vi "Teleop.vi"(10 "Match Info":T1={"Autonomous Elapsed Seconds"=0.0, "TeleOp Elapsed Seconds"=0.0, "Disabled Elapsed Seconds"=0.0, "Visited Autonomous"=FALSE, "Visited TeleOp"=FALSE, "Visited Disabled"=FALSE, "Autonomous Settings"={"Autonomous Style"=enum."Independent", "VI Refnum"=refnum}}, 11 "Call Context":T2) -> ()   [LabVIEW 2020]
doc: "This VI is called for each enabled TeleOp packet received from the DS. It is typically used to read from joysticks and other inputs and update I/O or setpoints for timed control loops. It should complete and return within 20 milliseconds or risk missing DS packets."
uses:
  <vilib>/Rock Robotics/Network Tables/NT Write Boolean Array.vi
  <vilib>/Rock Robotics/Network Tables/NT Write Numeric Array.vi
  Framework/Robot Global Data.vi
  <vilib>/Rock Robotics/WPI/DriverStation/WPI_DriverStationMatch Info.ctl
  <vilib>/Rock Robotics/WPI/DriverStation/WPI_DriverStationDerivedRobotMode.ctl
panel:
  in  "Duration(s)":dbl=3.0 format="%#_13g"
  in  "Shorter Setpoint":dbl=0.8 format="%#_13g"
  in  "Duration(s)":dbl=3.0 format="%#_13g"
  in  "Shorter Setpoint":dbl=0.8 format="%#_13g"
  in  "Duration(s)":dbl=3.0 format="%#_13g"
  in  "Shorter Setpoint":dbl=0.8 format="%#_13g"
  in  "Duration(s)":dbl=3.0 format="%#_13g"
  in  "Shorter Setpoint":dbl=0.8 format="%#_13g"
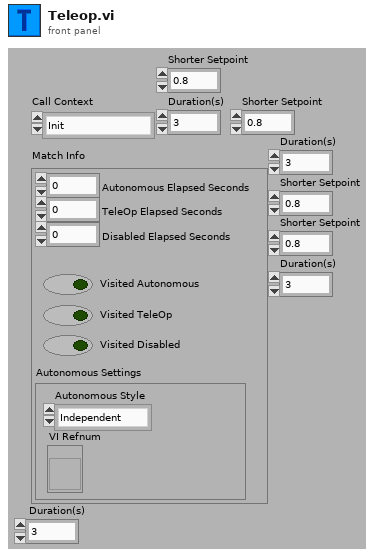
[diagram p1: front panel]
types:
  T1 = typedef "WPI_DriverStationMatch Info.ctl" = cluster{"Autonomous Elapsed Seconds":dbl, "TeleOp Elapsed Seconds":dbl, "Disabled Elapsed Seconds":dbl, "Visited Autonomous":bool, "Visited TeleOp":bool, "Visited Disabled":bool, "Autonomous Settings":cluster{"Autonomous Style":enum16{"Iterative", "Independent"}, "VI Refnum":refnum<vi>}}
  T2 = typedef "WPI_DriverStationDerivedRobotMode.ctl" = enum16{"Init", "Execute", "Stop"}
  T3 = typedef "WPI_JoystickDevRef.ctl" = cluster{"Device":T4}
  T4 = typedef "WPI_JoystickDeviceEnum.ctl" = enum16{"USB 0", "USB 1", "USB 2", "USB 3", "USB 4", "USB 5"}
  T5 = typedef "Command Status Info.ctl" = cluster{"Name":string, "Status":T6, "notifier out":T7}
  T6 = typedef "Completion Status.ctl" = enum16{"Successful", "Aborted", "Incomplete"}
  T7 = typedef "Completion Notifier.ctl" = refnum<notifier>
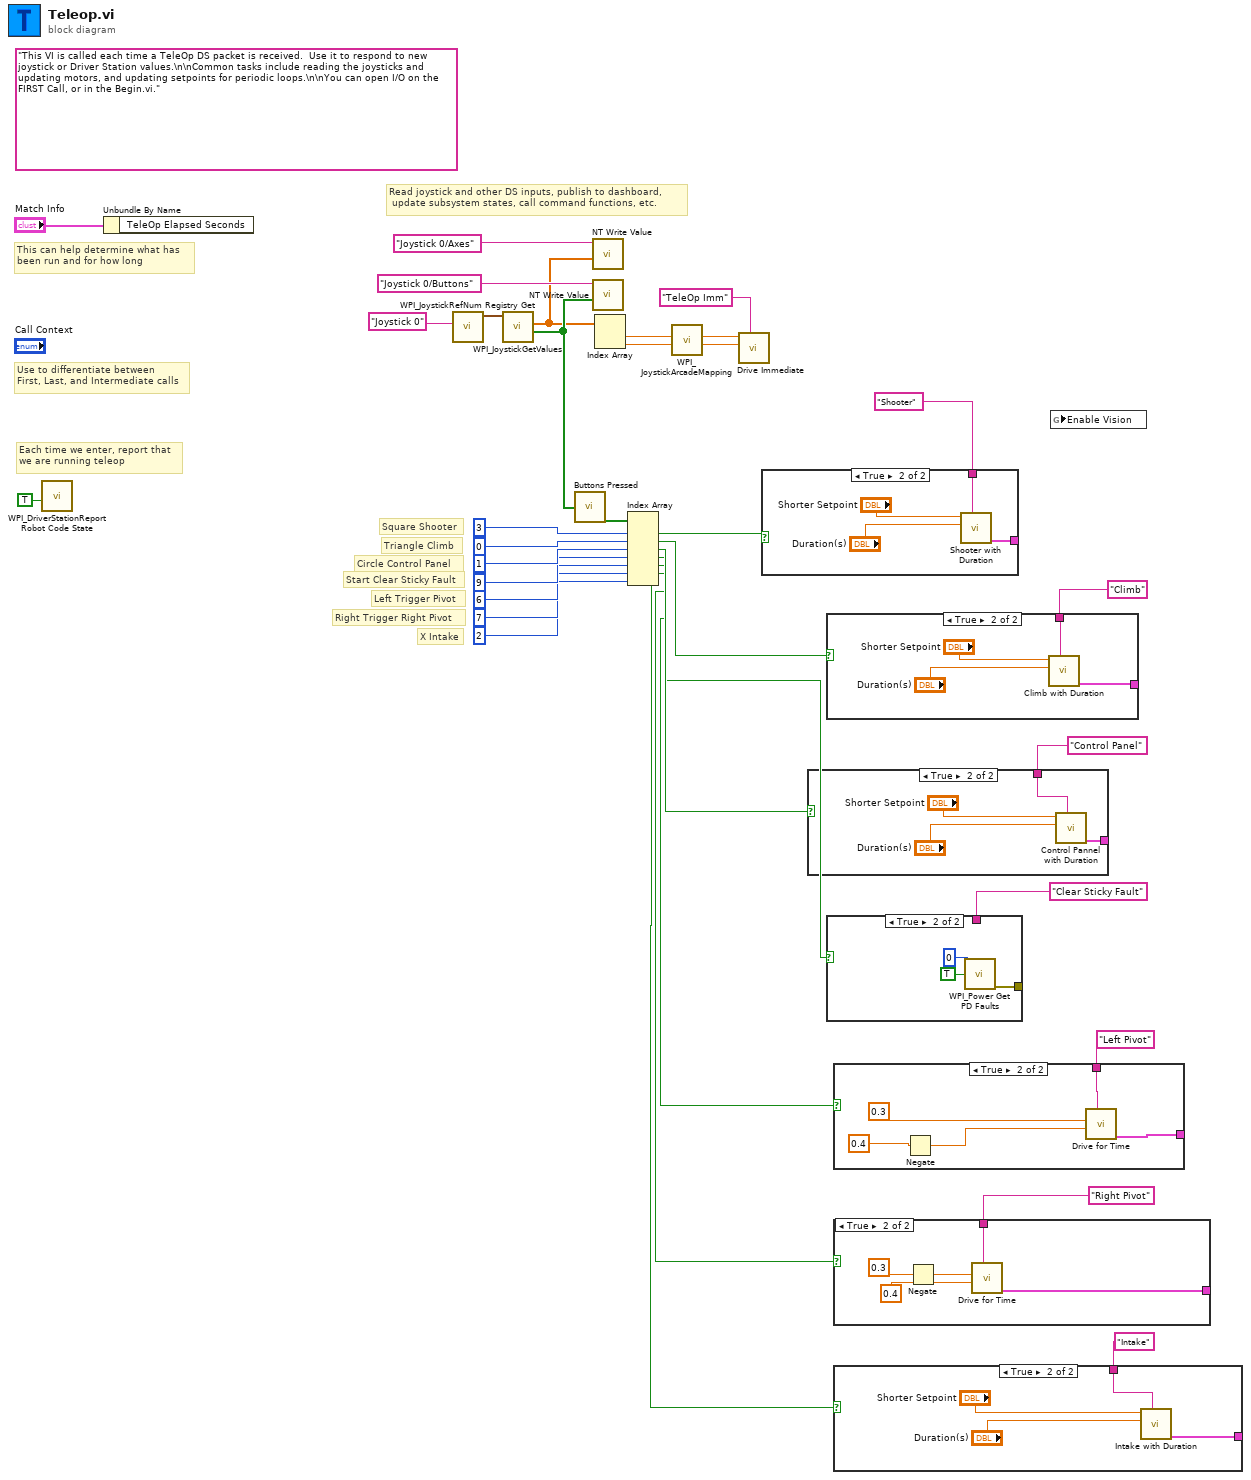
[diagram p0: block diagram]
diagram:
  (unwired) "This VI is called each time a TeleOp DS packet is received.  Use it to respond to new joystick or Driver Station values.\n\nCommon tasks include reading the joysticks and updating motors, and updating setpoints for periodic loops.\n\nYou can open I/O on the FIRST Call, or in the Begin.vi."
  # "X Intake"
  # "Right Trigger Right Pivot"
  # "Left Trigger Pivot"
  # "Start Clear Sticky Fault"
  # "Circle Control Panel"
  # "Triangle Climb"
  # "Square Shooter"
  # "Read joystick and other DS inputs, publish to dashboard,\n update subsystem states, call command functions, etc."
  # "Each time we enter, report that\nwe are running teleop"
  # "Use to differentiate between\nFirst, Last, and Intermediate calls"
  # "This can help determine what has\nbeen run and for how long"
  n1 = call <vilib>:"WPI_DriverStationReport Robot Code State.vi"("TeleOp"=TRUE ("Autonomous")) -> ()  [unwired: 10 in, 1 out]
  n2 = Unbundle By Name("Match Info") -> ()  [unwired: 1 out]
  n3 = call <vilib>:"WPI_JoystickRefNum Registry Get.vi"("refnum name"="Joystick 0") -> ("JoystickDevRef"=w32:T3)  [unwired: 1 in, 9 out]
  n4 = call <vilib>:"WPI_JoystickGetValues.vi"("JoystickDevRef"=w32) -> ("Buttons"=w20:bool[], "Axes"=w19:dbl[])  [unwired: 6 in, 3 out]
  n5 = call "Buttons Pressed.vi"("Button Values"=w20) -> ("Button Presses"=w28:bool[])
  n6 = call-poly <vilib>:"NT Write Value.vi"("Numeric Array"=w19, "Name"="Joystick 0/Axes") -> ()  [unwired: 9 in, 1 out]
  n7 = call-poly <vilib>:"NT Write Value.vi"("Boolean Array"=w20, "Name"="Joystick 0/Buttons") -> ()  [unwired: 9 in, 1 out]
  n8 = Index Array(array=w19) -> (element #1=w23:dbl, element #2=w22:dbl)  [unwired: 2 in]
  n9 = Index Array(array=w28, index #1=3 ("index"), index #2=0 ("index"), index #3=1 ("index"), index #4=9 ("index"), index #5=6 ("index"), index #6=7 ("index"), index #7=2 ("index")) -> (element #1=w27:bool, element #2=w26:bool, element #3=w5:bool, element #4=w4:bool, element #5=w3:bool, element #6=w2:bool, element #7=w1:bool)
  n10 = call <vilib>:"WPI_JoystickArcadeMapping.vi"("Y axis value"=w22, "X axis value"=w23) -> ("Right Motor Value"=w24:dbl, "Left Motor Value"=w25:dbl)  [unwired: 8 in]
  n11 = call "Drive Immediate.vi"("Description"="TeleOp Imm", "Right Setpoint"=w24, "Left Setpoint"=w25) -> ()  [unwired: 8 in, 1 out]
  n12 = case shown="True" w27 {
    tunnel: [_ w39] -> _
    tunnel: "Shooter" ("Description") -> [_ w38]
    frame False {
    }
    frame True {
      n13 = call "Shooter with Duration.vi"("Description"=w38, "Duration (s)"="Duration(s)", "Setpoint"="Shorter Setpoint") -> ("Command Info Out"=w39:T5)  [unwired: 8 in]
    }
  }
  n14 = case shown="True" w5 {
    tunnel: [_ w42] -> _
    tunnel: "Control Panel" ("Description") -> [_ w41]
    frame False {
    }
    frame True {
      n15 = call "Control Pannel with Duration.vi"("Description"=w41, "Duration (s)"="Duration(s)", "Setpoint"="Shorter Setpoint") -> ("Command Info Out"=w42:T5)  [unwired: 8 in]
    }
  }
  n16 = case shown="True" w26 {
    tunnel: [_ w46] -> _
    tunnel: "Climb" ("Description") -> [_ w45]
    frame False {
    }
    frame True {
      n17 = call "Climb with Duration.vi"("Description"=w45, "Duration (s)"="Duration(s)", "Setpoint"="Shorter Setpoint") -> ("Command Info Out"=w46:T5)  [unwired: 8 in]
    }
  }
  n18 = case shown="True" w4 {
    tunnel: [_ w50] -> _
    tunnel: "Clear Sticky Fault" ("Description") -> [_ _]
    frame False {
    }
    frame True {
      n19 = call <vilib>:"WPI_Power Get PD Faults.vi"("Power Distribution (def)"=u8 0, "Clear Sticky Faults"=TRUE) -> ("error out"=w50:errorcluster)  [unwired: 10 in, 3 out]
    }
  }
  n20 = case shown="True" w3 {
    tunnel: [_ w55] -> _
    tunnel: "Left Pivot" ("Description") -> [_ w54]
    frame False {
    }
    frame True {
      n21 = Negate(x=0.4) -> (-x=w51:dbl)
      n22 = call "Drive for Time.vi"("Description"=w54, "Seconds"=w51, "Right Speed"=0.3) -> ("Command Info Out"=w55:T5)  [unwired: 8 in]
    }
  }
  n23 = case shown="True" w2 {
    tunnel: [_ w59] -> _
    tunnel: "Right Pivot" ("Description") -> [_ w58]
    frame False {
    }
    frame True {
      n24 = Negate(x=0.3) -> (-x=w56:dbl)
      n25 = call "Drive for Time.vi"("Description"=w58, "Seconds"=0.4, "Right Speed"=w56) -> ("Command Info Out"=w59:T5)  [unwired: 8 in]
    }
  }
  n26 = case shown="True" w1 {
    tunnel: [_ w62] -> _
    tunnel: "Intake" ("Description") -> [_ w61]
    frame False {
    }
    frame True {
      n27 = call "Intake with Duration.vi"("Description"=w61, "Duration (s)"="Duration(s)", "Setpoint"="Shorter Setpoint") -> ("Command Info Out"=w62:T5)  [unwired: 8 in]
    }
  }
  n28 = global read "Robot Global Data.vi" "Enable Vision"() -> ()  [unwired: 1 in]
